vi "AFM_Driver_Manager.SetActive.vi"(8 "error in (no error)":errorcluster, 10 "Active Index":i32, 11 "AFM_Driver_Manager in":refnum<class "AFM_Driver_Manager.lvclass">) -> (0 "error out":errorcluster, 3 "AFM_Driver_Manager out":refnum<class "AFM_Driver_Manager.lvclass">)   [LabVIEW 2019, in "AFM_Driver_Manager.lvclass"]
uses:
  AFM_Driver_Manager.lvclass
  AFM_Driver_Manager.lvclass/AFM_Driver_Manager.ctl
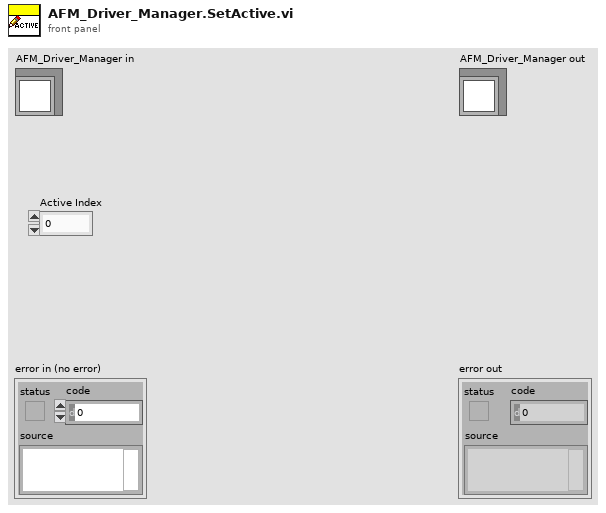
[diagram p1: front panel]
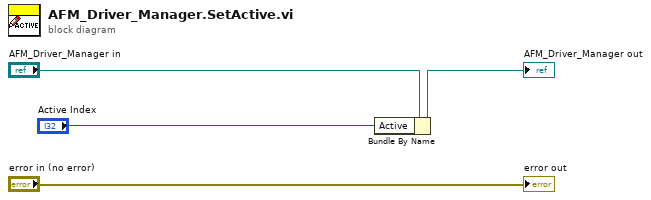
[diagram p0: block diagram]
diagram:
  n1 = Bundle By Name(cluster="AFM_Driver_Manager in", "Active"="Active Index") -> (→"AFM_Driver_Manager out":refnum<class "AFM_Driver_Manager.lvclass">)
  "error out" <- "error in (no error)"
